vi "RT Host - normalised speed profile.vi"(7 "Which speed profile?":T1, 8 "Error In":errorcluster, 11 "X input (normalised 0-1)":dbl) -> (0 "Error Out":errorcluster, 2 "Profile Mean":dbl format="%0.2f", 3 "Y output (normalised 0-1)":dbl)   [LabVIEW 2017]
doc: "This subVI provides a Y-value according to a defined x-input by interpolating a senables multiple normailsed profiles to be created and followed according to."
uses:
  Controls/hCAAR - speed profile.ctl
  <vilib>/Analysis/1siggen.llb/Ramp Pattern by Samples.vi
  <vilib>/Analysis/baseanly.llb/Mean (DBL).vi
  <vilib>/Analysis/NI_AALPro.lvlib
  <vilib>/Analysis/NI_AALBase.lvlib
panel:
  out "Speed Profile":cluster{dbl[], "Interpolant":dbl[]}(graph)={[0.0, 0.010101010101010102, 0.020202020202020204, 0.030303030303030304, 0.04040404040404041, 0.050505050505050504, 0.06060606060606061, 0.0707070707070707, 0.08080808080808081, 0.09090909090909091, 0.10101010101010101, 0.1111111111111111, 0.12121212121212122, 0.13131313131313133, 0.1414141414141414, 0.15151515151515152, 0.16161616161616163, 0.1717171717171717, 0.18181818181818182, 0.1919191919191919, 0.20202020202020202, 0.21212121212121213, 0.2222222222222222, 0.23232323232323232, 0.24242424242424243, 0.25252525252525254, 0.26262626262626265, 0.2727272727272727, 0.2828282828282828, 0.29292929292929293, 0.30303030303030304, 0.31313131313131315, 0.32323232323232326, 0.3333333333333333, 0.3434343434343434, 0.35353535353535354, 0.36363636363636365, 0.37373737373737376, 0.3838383838383838, 0.3939393939393939, 0.40404040404040403, 0.41414141414141414, 0.42424242424242425, 0.43434343434343436, 0.4444444444444444, 0.45454545454545453, 0.46464646464646464, 0.47474747474747475, 0.48484848484848486, 0.494949494949495, 0.5050505050505051, 0.5151515151515151, 0.5252525252525253, 0.5353535353535354, 0.5454545454545454, 0.5555555555555556, 0.5656565656565656, 0.5757575757575758, 0.5858585858585859, 0.5959595959595959, 0.6060606060606061, 0.6161616161616161, 0.6262626262626263, 0.6363636363636364, 0.6464646464646465, 0.6565656565656566, 0.6666666666666666, 0.6767676767676768, 0.6868686868686869, 0.696969696969697, 0.7070707070707071, 0.7171717171717171, 0.7272727272727273, 0.7373737373737373, 0.7474747474747475, 0.7575757575757576, 0.7676767676767676, 0.7777777777777778, 0.7878787878787878, 0.797979797979798, 0.8080808080808081, 0.8181818181818182, 0.8282828282828283, 0.8383838383838383, 0.8484848484848485, 0.8585858585858586, 0.8686868686868687, 0.8787878787878788, 0.8888888888888888, 0.898989898989899, 0.9090909090909091, 0.9191919191919192, 0.9292929292929293, 0.9393939393939394, 0.9494949494949495, 0.9595959595959596, 0.9696969696969697, 0.9797979797979798, 0.98989898989899, 1.0], "Interpolant"=[0.0, 0.03141075907812829, 0.06279051952931337, 0.09410831331851431, 0.12533323356430423, 0.15643446504023087, 0.1873813145857246, 0.21814324139654254, 0.24868988716485477, 0.2789911060392292, 0.3090169943749474, 0.33873792024529137, 0.3681245526846779, 0.3971478906347806, 0.4257792915650726, 0.4539904997395468, 0.4817536741017152, 0.5090414157503713, 0.5358267949789965, 0.5620833778521306, 0.587785252292473, 0.6129070536529765, 0.6374239897486896, 0.6613118653236518, 0.6845471059286886, 0.7071067811865475, 0.7289686274214114, 0.7501110696304595, 0.7705132427757891, 0.7901550123756903, 0.8090169943749473, 0.8270805742745617, 0.844327925502015, 0.8607420270039435, 0.8763066800438635, 0.8910065241883678, 0.9048270524660195, 0.917754625683981, 0.9297764858882513, 0.9408807689542253, 0.9510565162951535, 0.960293685676943, 0.9685831611286311, 0.9759167619387473, 0.9822872507286886, 0.9876883405951377, 0.9921147013144778, 0.99556196460308, 0.9980267284282716, 0.9995065603657316, 1.0, 0.9995065603657316, 0.9980267284282716, 0.9955619646030801, 0.9921147013144779, 0.9876883405951379, 0.9822872507286887, 0.9759167619387475, 0.9685831611286312, 0.9602936856769432, 0.9510565162951536, 0.9408807689542256, 0.9297764858882515, 0.9177546256839813, 0.9048270524660196, 0.891006524188368, 0.8763066800438637, 0.8607420270039438, 0.8443279255020152, 0.8270805742745619, 0.8090169943749476, 0.7901550123756905, 0.7705132427757894, 0.7501110696304597, 0.7289686274214117, 0.7071067811865477, 0.6845471059286888, 0.661311865323652, 0.6374239897486899, 0.6129070536529767, 0.5877852522924732, 0.5620833778521308, 0.5358267949789968, 0.5090414157503715, 0.48175367410171543, 0.453990499739547, 0.4257792915650728, 0.39714789063478084, 0.36812455268467814, 0.3387379202452916, 0.3090169943749476, 0.27899110603922944, 0.248689887164855, 0.21814324139654273, 0.18738131458572485, 0.15643446504023106, 0.12533323356430448, 0.09410831331851452, 0.06279051952931362, 0.03141075907812849]}
  in  "User-Defined":cluster{"X":dbl, "Y":dbl}[](array[cluster])=[{"X"=0.0, "Y"=0.0}, {"X"=0.0600000000000001, "Y"=0.13000000000000006}, {"X"=0.10999999999999996, "Y"=0.2999999999999998}, {"X"=0.17999999999999988, "Y"=0.5299999999999998}, {"X"=0.33999999999999997, "Y"=0.8599999999999999}, {"X"=0.47, "Y"=0.98}, {"X"=0.61, "Y"=0.99}, {"X"=0.8, "Y"=0.8600000000000001}, {"X"=0.8800000000000001, "Y"=0.5800000000000001}, {"X"=0.9500000000000001, "Y"=0.19000000000000006}, {"X"=1.0, "Y"=0.0}] {"Y" step=0.01; "X" step=0.01}
  # "Outputs"
  # "Inputs"
  # "Local Data"
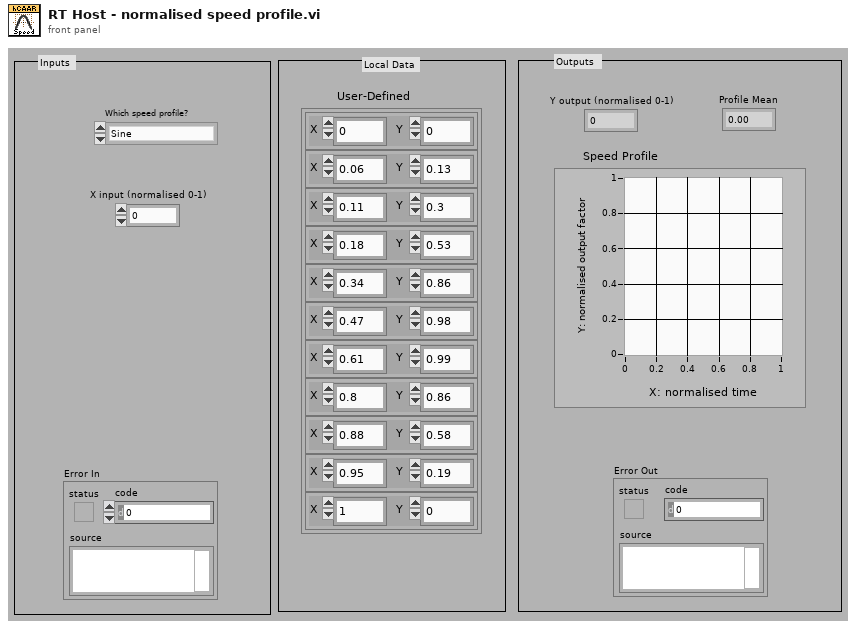
[diagram p1: front panel]
types:
  T1 = typedef "hCAAR - speed profile.ctl" = enum16{"Sine", "Sine With Initial Shunt", "Triangle", "Square", "Sawtooth", "Forward Skew", "User Defined"}
  T2 = enum16{"sine", "cosine", "triangle", "square", "sawtooth", "increasing ramp", "decreasing ramp"}
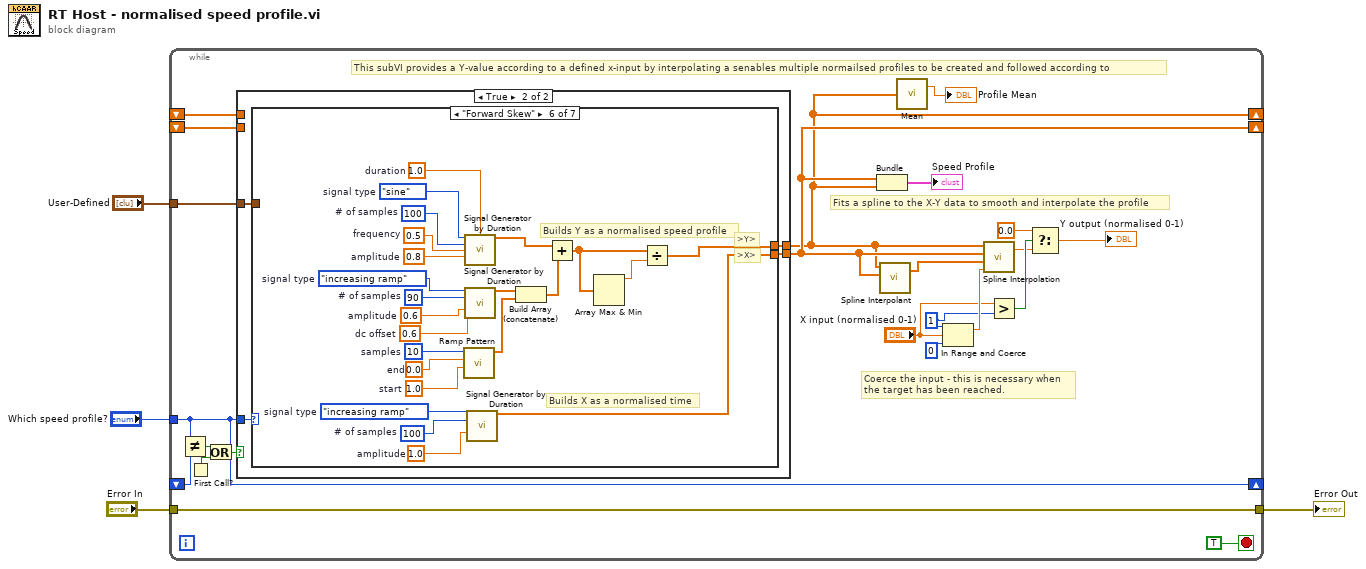
[diagram p0: block diagram]
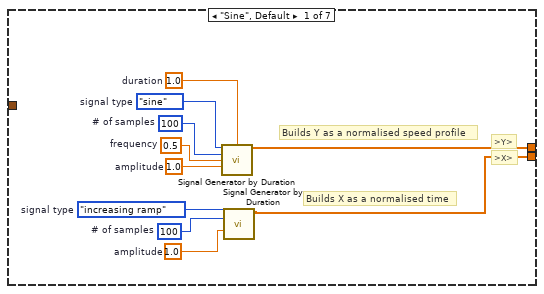
[diagram p3: hidden frame]
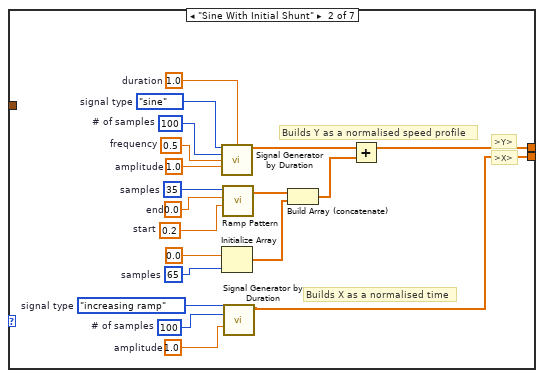
[diagram p4: hidden frame]
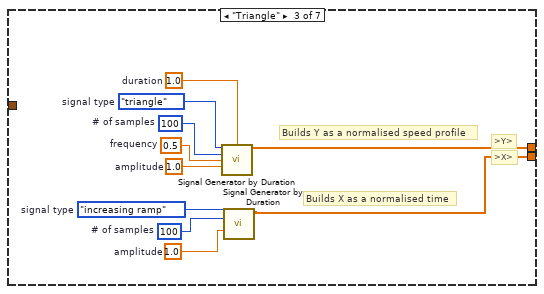
[diagram p5: hidden frame]
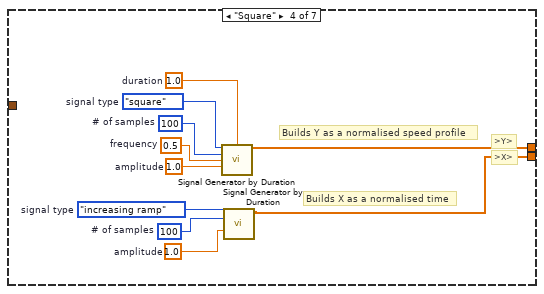
[diagram p6: hidden frame]
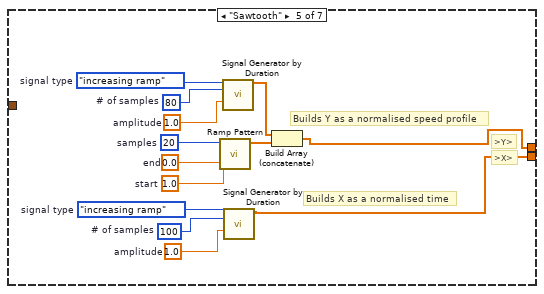
[diagram p7: hidden frame]
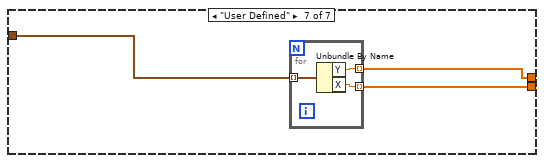
[diagram p8: hidden frame]
diagram:
  n1 = while {
    tunnel: "User-Defined" -> [w27]
    tunnel: "Which speed profile?" -> [w12]
    tunnel: [w16] -> w2
    tunnel: "Error In" -> [w16]
    shift-right: [w9] -> _
    shift-left: _ -> [w14]
    shift-right: [w10] -> _
    shift-left: _ -> [w13]
    shift-right: [w12] -> _
    shift-left: _ -> [w11]
    stop <- TRUE stop-if-true
    w24 = 1
    # "This subVI provides a Y-value according to a defined x-input by interpolating a senables multiple normailsed profiles to be created and followed according to"
    # "Fits a spline to the X-Y data to smooth and interpolate the profile"
    # "Coerce the input - this is necessary when\nthe target has been reached."
    n2 = Not Equal?(x=w12, y=w11) -> (x != y?=w7:bool)
    n3 = First Call?() -> (First Call?: T/F=w5:bool)
    n4 = Or(x=w7, y=w5) -> (x .or. y?=w6:bool)
    n5 = case shown="True" w6 {
      tunnel: w27 -> [_ w33]
      tunnel: w12 -> [_ w32]
      tunnel: [w28 w31] -> w10
      tunnel: [w29 w30] -> w9
      tunnel: w14 -> [w29 _]
      tunnel: w13 -> [w28 _]
      frame False {
        # "Saves CPU by only generating a new profile array when the profile type is changed"
      }
      frame True {
        n6 = case shown="\"Forward Skew\"" w32 {
          tunnel: [w34 w53 w63 w73 w92 w110 w121] -> w31
          tunnel: [w38 w45 w67 w77 w87 w97 w119] -> w30
          tunnel: w33 -> [_ _ _ _ _ _ w120]
          frame "Sine", Default {
            w36 = 100  # # of samples
            w35 = 1.0  # amplitude
            w37 = T2."increasing ramp"  # signal type
            w39 = 1.0  # duration
            w40 = 100  # # of samples
            w41 = 0.5  # frequency
            w42 = 1.0  # amplitude
            w43 = T2."sine"  # signal type
            # "Builds Y as a normalised speed profile"
            # "Builds X as a normalised time"
            # ">X>"
            # ">Y>"
            n7 = call <vilib>:"Signal Generator by Duration.vi"("signal type"=w43, "duration"=w39, "# of samples"=w40, "frequency"=w41, "amplitude"=w42) -> ("signal"=w38:dbl[])  [unwired: 7 in, 3 out]
            n8 = call <vilib>:"Signal Generator by Duration.vi"("signal type"=w37, "# of samples"=w36, "amplitude"=w35) -> ("signal"=w34:dbl[])  [unwired: 9 in, 3 out]
          }
          frame "Sine With Initial Shunt" {
            w51 = 65  # samples
            w46 = 0.2  # start
            w48 = 0.0  # end
            w47 = 35  # samples
            w55 = 100  # # of samples
            w54 = 1.0  # amplitude
            w56 = T2."increasing ramp"  # signal type
            w58 = 1.0  # duration
            w59 = 100  # # of samples
            w60 = 0.5  # frequency
            w61 = 1.0  # amplitude
            w62 = T2."sine"  # signal type
            # "Builds Y as a normalised speed profile"
            # "Builds X as a normalised time"
            # ">X>"
            # ">Y>"
            n9 = call <vilib>:"Signal Generator by Duration.vi"("signal type"=w62, "duration"=w58, "# of samples"=w59, "frequency"=w60, "amplitude"=w61) -> ("signal"=w57:dbl[])  [unwired: 7 in, 3 out]
            n10 = Initialize Array(0.0 ("element"), w51) -> (w52:dbl[])
            n11 = call-poly <vilib>:"Ramp Pattern.vi"("start"=w46, "end"=w48, "samples"=w47) -> ("Ramp Pattern"=w49:dbl[])  [unwired: 7 in, 1 out]
            n12 = call <vilib>:"Signal Generator by Duration.vi"("signal type"=w56, "# of samples"=w55, "amplitude"=w54) -> ("signal"=w53:dbl[])  [unwired: 9 in, 3 out]
            n13 = Build Array (concatenate)(w49, w52) -> (w44:dbl[])
            n14 = Add(x=w57, y=w44) -> (x+y=w45:dbl[])
          }
          frame "Triangle" {
            w65 = 100  # # of samples
            w64 = 1.0  # amplitude
            w66 = T2."increasing ramp"  # signal type
            w68 = 1.0  # duration
            w69 = 100  # # of samples
            w70 = 0.5  # frequency
            w71 = 1.0  # amplitude
            w72 = T2."triangle"  # signal type
            # "Builds Y as a normalised speed profile"
            # "Builds X as a normalised time"
            # ">X>"
            # ">Y>"
            n15 = call <vilib>:"Signal Generator by Duration.vi"("signal type"=w72, "duration"=w68, "# of samples"=w69, "frequency"=w70, "amplitude"=w71) -> ("signal"=w67:dbl[])  [unwired: 7 in, 3 out]
            n16 = call <vilib>:"Signal Generator by Duration.vi"("signal type"=w66, "# of samples"=w65, "amplitude"=w64) -> ("signal"=w63:dbl[])  [unwired: 9 in, 3 out]
          }
          frame "Square" {
            w75 = 100  # # of samples
            w74 = 1.0  # amplitude
            w76 = T2."increasing ramp"  # signal type
            w78 = 1.0  # duration
            w79 = 100  # # of samples
            w80 = 0.5  # frequency
            w81 = 1.0  # amplitude
            w82 = T2."square"  # signal type
            # "Builds Y as a normalised speed profile"
            # "Builds X as a normalised time"
            # ">X>"
            # ">Y>"
            n17 = call <vilib>:"Signal Generator by Duration.vi"("signal type"=w82, "duration"=w78, "# of samples"=w79, "frequency"=w80, "amplitude"=w81) -> ("signal"=w77:dbl[])  [unwired: 7 in, 3 out]
            n18 = call <vilib>:"Signal Generator by Duration.vi"("signal type"=w76, "# of samples"=w75, "amplitude"=w74) -> ("signal"=w73:dbl[])  [unwired: 9 in, 3 out]
          }
          frame "Sawtooth" {
            w83 = 1.0  # start
            w84 = 0.0  # end
            w85 = 20  # samples
            w90 = 80  # # of samples
            w91 = 1.0  # amplitude
            w89 = T2."increasing ramp"  # signal type
            w94 = 100  # # of samples
            w93 = 1.0  # amplitude
            w95 = T2."increasing ramp"  # signal type
            # "Builds Y as a normalised speed profile"
            # "Builds X as a normalised time"
            # ">X>"
            # ">Y>"
            n19 = call-poly <vilib>:"Ramp Pattern.vi"("start"=w83, "end"=w84, "samples"=w85) -> ("Ramp Pattern"=w86:dbl[])  [unwired: 7 in, 1 out]
            n20 = call <vilib>:"Signal Generator by Duration.vi"("signal type"=w89, "# of samples"=w90, "amplitude"=w91) -> ("signal"=w88:dbl[])  [unwired: 9 in, 3 out]
            n21 = call <vilib>:"Signal Generator by Duration.vi"("signal type"=w95, "# of samples"=w94, "amplitude"=w93) -> ("signal"=w92:dbl[])  [unwired: 9 in, 3 out]
            n22 = Build Array (concatenate)(w88, w86) -> (w87:dbl[])
          }
          frame "Forward Skew" {
            w96 = 0.6  # dc offset
            w101 = 1.0  # start
            w103 = 0.0  # end
            w102 = 10  # samples
            w108 = 90  # # of samples
            w109 = 0.6  # amplitude
            w107 = T2."increasing ramp"  # signal type
            w112 = 100  # # of samples
            w111 = 1.0  # amplitude
            w113 = T2."increasing ramp"  # signal type
            w114 = 1.0  # duration
            w115 = 100  # # of samples
            w116 = 0.5  # frequency
            w117 = 0.8  # amplitude
            w118 = T2."sine"  # signal type
            # "Builds Y as a normalised speed profile"
            # "Builds X as a normalised time"
            # ">X>"
            # ">Y>"
            n23 = call-poly <vilib>:"Ramp Pattern.vi"("start"=w101, "end"=w103, "samples"=w102) -> ("Ramp Pattern"=w100:dbl[])  [unwired: 7 in, 1 out]
            n24 = call <vilib>:"Signal Generator by Duration.vi"("signal type"=w118, "duration"=w114, "# of samples"=w115, "frequency"=w116, "amplitude"=w117) -> ("signal"=w106:dbl[])  [unwired: 7 in, 3 out]
            n25 = call <vilib>:"Signal Generator by Duration.vi"("signal type"=w107, "# of samples"=w108, "amplitude"=w109, "dc offset"=w96) -> ("signal"=w105:dbl[])  [unwired: 8 in, 3 out]
            n26 = call <vilib>:"Signal Generator by Duration.vi"("signal type"=w113, "# of samples"=w112, "amplitude"=w111) -> ("signal"=w110:dbl[])  [unwired: 9 in, 3 out]
            n27 = Build Array (concatenate)(w105, w100) -> (w104:dbl[])
            n28 = Add(x=w106, y=w104) -> (x+y=w98:dbl[])
            n29 = Array Max & Min(array=w98) -> (max value=w99:dbl)  [unwired: 3 out]
            n30 = Divide(x=w98, y=w99) -> (x/y=w97:dbl[])
          }
          frame "User Defined" {
            n31 = for {
              tunnel: w120 -> [w124] mode=indexing
              tunnel: [w123] -> w119 mode=indexing
              tunnel: [w122] -> w121 mode=indexing
              n32 = Unbundle By Name(w124) -> ("Y"=w123:dbl, "X"=w122:dbl)
            }
          }
        }
      }
    }
    n33 = Bundle("signal"=w10, "signal"=w9) -> (→"Speed Profile":cluster{"signal":dbl[], "signal":dbl[]})  [unwired: 1 in]
    n34 = call <vilib>:"Spline Interpolant.vi"("X"=w10, "Y"=w9) -> ("Interpolant"=w18:dbl[])  [unwired: 2 in, 1 out]
    n35 = call-poly <vilib>:"Mean.vi"("X"=w9) -> ("mean"=→"Profile Mean":dbl)  [unwired: 1 out]
    n36 = In Range and Coerce(upper limit=w24, x="X input (normalised 0-1)", lower limit=0) -> (coerced(x)=w25:dbl)  [unwired: 1 out]
    n37 = call <vilib>:"Spline Interpolation.vi"("x value"=w25, "Interpolant"=w18, "X"=w10, "Y"=w9) -> ("interpolation value"=w20:dbl)  [unwired: 1 out]
    n38 = Greater?(x="X input (normalised 0-1)", y=w24) -> (0:w21:bool)
    n39 = Select(t=0.0, s=w21, f=w20) -> (s? t:f=→"Y output (normalised 0-1)":dbl)
  }
  "Error Out" <- w2
